vi "Decimation.vi"(9 "Samples per Symbol":i32, 11 "Signal In":cdb[](array[numeric])) -> (3 "Signal Out":cdb[](array[numeric]))   [LabVIEW 2011]
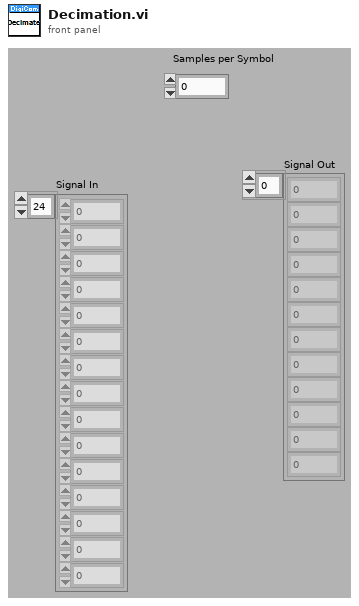
[diagram p1: front panel]
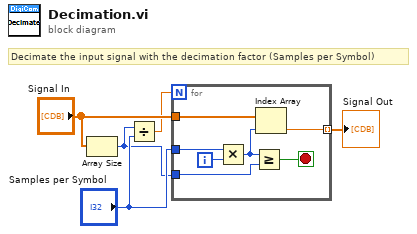
[diagram p0: block diagram]
diagram:
  # "Decimate the input signal with the decimation factor (Samples per Symbol)"
  n1 = Array Size(array="Signal In") -> (size(s)=w2:i32)
  n2 = Divide(x=w2, y="Samples per Symbol") -> (x/y=w1:dbl)
  n3 = for {
    N: w1 -> [_]
    tunnel: "Samples per Symbol" -> [w12]
    tunnel: [w10] -> w5 mode=indexing
    tunnel: "Signal In" -> [w9]
    tunnel: w2 -> [w7]
    i -> [w11]
    stop <- w6 stop-if-true
    n4 = Multiply(x=w12, y=w11) -> (x*y=w8:i32)
    n5 = Greater Or Equal?(x=w8, y=w7) -> (x >= y?=w6:bool)
    n6 = Index Array(array=w9, index=w8) -> (element=w10:cdb)
  }
  "Signal Out" <- w5
